vi "PH_PSDBWriter.PSDBThread.vi"(0 "object ref":refnum<vi>, 5 "error in (no error)":errorcluster) -> (19 "error out":errorcluster)   [LabVIEW 2014, in "PH_PSDBWriter.lvlib"]
doc: "This Template-VI contains a loop to exchange data with the PSDB on request.\n\n\nLicense Agreement for this software:\n\nCopyright (C)\nGesellschaft für Schwerionenforschung, GSI\nPlanckstr. 1\n64291 Darmstadt\nGermany\n\nContact: H.Brand@gsi.de \n\nThis program is free software; you can redistribute it and/or modify it under the terms of the \nGNU General Public License as published by the Free Software Foundation; either version 2 of \nthe license, or (at your option) any later version.\n\nThis program is distributed in the hope that it will be useful, but WITHOUT ANY WARRANTY; \nwithout even the implied warranty of MERCHANTABILITY or FITNESS FOR A PARTICULAR PURPOSE. See \nthe GNU General License for more details (http://www.gnu.org).\n\nGesellschaft für Schwerionenforschung, GSI\nPlanckstr. 1, 64291 Darmstadt, Germany\nFor all questions and ideas contact: M.Richter@gsi.de, H.Brand@gsi.de or D.Beck@gsi.de.\nLast update: 13-JAN-2005"
uses:
  PH_PSDBWriter.lvlib
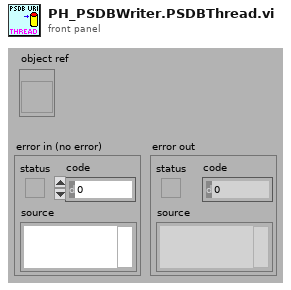
[diagram p1: front panel]
types:
  T1 = typedef "PH_PSDBWriter.lvlib/PH_PSDBWriter.i attribute.ctl" = cluster{"PSDB Status Service ID":i32, "Instance ID":i32, "Shot #":i32, "Subsystem":T2, "Data Status":T3, "Ref PSDB Status":refnum<vi>, "PSDB Error Code":i32, "PSDB Dataset":T4, "PSDB Thread":cluster{"Ref":refnum<vi>, "Q-Ref":refnum<queue>}, "PSDB Credentials":T12}
  T2 = typedef "PH_PSDBWriter.lvlib/PH_PSDBWriter.PHELIX-Subsystems.ctl" = i32
  T3 = typedef "PH_PSDBWriter.lvlib/PH_PSDBWriter.Data Status.ctl" = i16
  T4 = typedef "PH_PSDBWriter.lvlib/PH_PSDBWriter.PSDB Dataset.ctl" = cluster{"Version":i32, "2D data Input":T5[], "Boolean Input":T7[], "Image Input":T8[], "Numeric Input":T10[], "String Input":T11[]}
  T5 = typedef "PH_PSDBWriter.lvlib/PH_PSDBWriter.2D dataset.ctl" = cluster{"name":string, "data":dbl[][], "axis description":T6}
  T6 = typedef "PSDB.lvlib/PSDB_AxisDescription.ctl" = cluster{"x axis label":string, "y axis label":string, "x axis unit":string, "y axis unit":string}
  T7 = typedef "PH_PSDBWriter.lvlib/PH_PSDBWriter.Boolean dataset.ctl" = cluster{"name":string, "data":bool, "unit":string}
  T8 = typedef "PH_PSDBWriter.lvlib/PH_PSDBWriter.Image dataset.ctl" = cluster{"name":string, "data":T9, "unit":string}
  T9 = typedef "IMAQ Image.ctl" = refnum<image>
  T10 = typedef "PH_PSDBWriter.lvlib/PH_PSDBWriter.Numeric dataset.ctl" = cluster{"name":string, "data":dbl, "unit":string}
  T11 = typedef "PH_PSDBWriter.lvlib/PH_PSDBWriter.String dataset.ctl" = cluster{"name":string, "data":string, "unit":string}
  T12 = typedef "PH_Common.lvlib/PH_Connection.PSDB Credentials.ctl" = cluster{"PW":string, "ID":string, "DS":string}
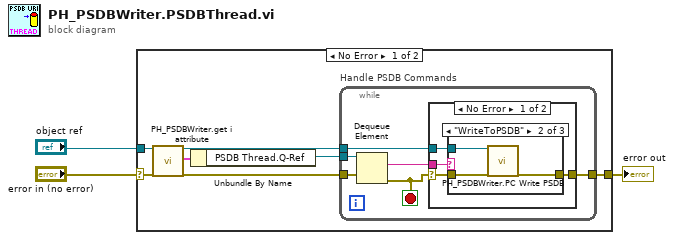
[diagram p0: block diagram]
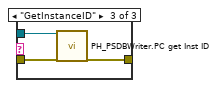
[diagram p3: hidden frame]
diagram:
  n1 = case shown="No Error" "error in (no error)" {
    selector: "error in (no error)" -> [w8 w29]
    tunnel: "object ref" -> [w10 _]
    tunnel: [w4 w29] -> w2
    frame No Error {
      n2 = call "PH_PSDBWriter.get i attribute.vi"("i ref in"=w10, "error in (no error)"=w8) -> ("i ref out"=w9:refnum<vi>, "i attribute"=w6:T1, "error out"=w7:errorcluster)  [unwired: 15 in]
      n3 = Unbundle By Name(w6) -> ("PSDB Thread.Q-Ref"=w5:refnum<queue>)
      n4 = while "Handle PSDB Commands" {
        tunnel: w9 -> [w16]
        tunnel: w7 -> [w14]
        tunnel: w5 -> [w15]
        tunnel: [w11] -> w4
        stop <- w13 stop-if-true
        n5 = Dequeue Element(queue=w15, error in (no error)=w14) -> (element=w12:string, error out=w13:errorcluster)  [unwired: 1 in, 2 out]
        n6 = case shown="No Error" w13 {
          selector: w13 -> [w19 w28]
          tunnel: w16 -> [w20 _]
          tunnel: w12 -> [w18 _]
          tunnel: [w17 w28] -> w11
          frame No Error {
            n7 = case shown="\"WriteToPSDB\"" w18 {
              tunnel: w20 -> [_ w24 w27]
              tunnel: w19 -> [w21 w23 w26]
              tunnel: [w21 w22 w25] -> w17
              frame Default {
              }
              frame "WriteToPSDB" {
                n8 = call "PH_PSDBWriter.PC Write PSDB.vi"("i ref in"=w24, "error IO"=w23) -> ("error out"=w22:errorcluster)  [unwired: 16 in, 1 out]
              }
              frame "GetInstanceID" {
                n9 = call "PH_PSDBWriter.PC get Inst ID.vi"("VI in"=w27, "error in (no error)"=w26) -> ("error out"=w25:errorcluster)  [unwired: 16 in, 1 out]
              }
            }
          }
          frame Error {
          }
        }
      }
    }
    frame Error {
    }
  }
  "error out" <- w2
